vi "setCleanCount.vi"(8 "error in (no error)":errorcluster, 10 "count":i32, 11 "CCD in":refnum<class "CCD.lvclass">) -> (0 "error out":errorcluster, 1 "ID":i32, 2 "results-JSON string":string, 3 "CCD out":refnum<class "CCD.lvclass">)   [LabVIEW 2023, in "CCD.lvclass"]
uses:
  CCD.lvclass
  CCD.lvclass/CCD.ctl
  20f7d3bd-08ac-4524-9bed-df36c1da25a0.vi
  GenericDevice/GenericDevice.lvclass
  cab240a6-cbf4-4e2c-ab79-96d9c1b88265.vi
  <vilib>/IlluminatedG/lv-web-crypto/lv-json/JSON/JSON.lvlib
  28418afd-abcd-4dad-a3f7-ef0ce47be2ad.vi
panel:
  in  "mode":i32
  # "Connector Pane"
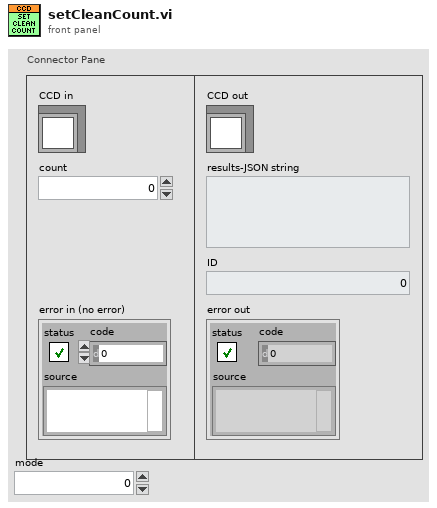
[diagram p1: front panel]
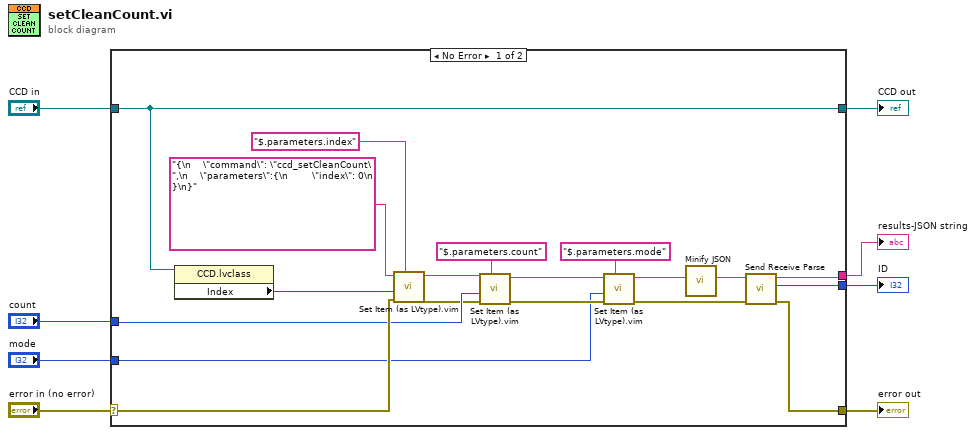
[diagram p0: block diagram]
diagram:
  n1 = case shown="No Error" "error in (no error)" {
    selector: "error in (no error)" -> [w23 w29]
    tunnel: [w18 w29] -> w7
    tunnel: [w25 w28] -> w5
    tunnel: "CCD in" -> [w25 w28]
    tunnel: "count" -> [w21 _]
    tunnel: [w17 _] -> w4
    tunnel: [w16 _] -> w3
    tunnel: "mode" -> [w9 _]
    frame No Error {
      n2 = property class="CCD.lvclass"(reference=w25) -> ("Index"=w24:i32)  [unwired: 1 in, 2 out]
      n3 = call "Set Item (as LVtype).vim"("$Path or Item Name"="$.parameters.index", "error in (no error)"=w23, "Anything"=w24, "JSON"="{\n    \"command\": \"ccd_setCleanCount\",\n    \"parameters\":{\n        \"index\": 0\n    }\n}") -> ("error out"=w20:errorcluster, "<JSON>"=w19:string)  [unwired: 4 in, 1 out]
      n4 = call "Set Item (as LVtype).vim"("$Path or Item Name"="$.parameters.count", "error in (no error)"=w20, "Anything"=w21, "JSON"=w19) -> ("error out"=w11:errorcluster, "<JSON>"=w13:string)  [unwired: 4 in, 1 out]
      n5 = call "Set Item (as LVtype).vim"("$Path or Item Name"="$.parameters.mode", "error in (no error)"=w11, "Anything"=w9, "JSON"=w13) -> ("error out"=w10:errorcluster, "<JSON>"=w12:string)  [unwired: 4 in, 1 out]
      n6 = call <vilib>:"Minify JSON.vi"("JSON String"=w12) -> ("Minified JSON"=w15:string)  [unwired: 10 in]
      n7 = call "Send Receive Parse.vi"("error in"=w10, "<JSON>"=w15) -> ("error out"=w18:errorcluster, "ID"=w16:i32, "results-JSON string"=w17:string)  [unwired: 7 in]
    }
    frame Error {
    }
  }
  "error out" <- w7
  "CCD out" <- w5
  "results-JSON string" <- w4
  "ID" <- w3
